vi "ELVIS III v1.0 Build MUX Configuration AO.vi"(11 "AO Channels List":T4) -> (3 "Channel Reservation Info":T1)   [LabVIEW 2021]
uses:
  <vilib>/myRIO/Common/Instrument Driver Framework/myRIO v1.0/AO/typedefs/AO Channels List.ctl
  <vilib>/myRIO/Common/Instrument Driver Framework/myRIO v1.0/AO/typedefs/AO Channels Enum.ctl
  <vilib>/myRIO/Common/Instrument Driver Framework/ELVIS III v1.0/Resource Manager/typedefs/ELVIS III v1.0 Channel Reservation List.ctl
  <vilib>/myRIO/Common/Instrument Driver Framework/ELVIS III v1.0/Resource Manager/typedefs/ELVIS III v1.0 Channel Reservation Info.ctl
  <vilib>/myRIO/Common/Instrument Driver Framework/ELVIS III v1.0/Resource Manager/typedefs/ELVIS III v1.0 Connector List.ctl
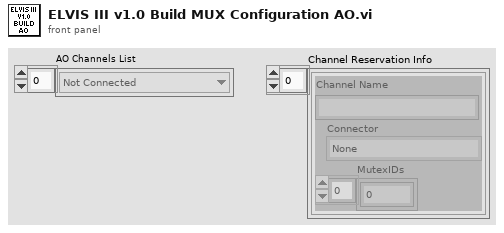
[diagram p1: front panel]
types:
  T1 = typedef "ELVIS III v1.0 Channel Reservation List.ctl" = T2[]
  T2 = typedef "ELVIS III v1.0 Channel Reservation Info.ctl" = cluster{"Channel Name":string, "Connector":T3, "MutexIDs":u32[]}
  T3 = typedef "ELVIS III v1.0 Connector List.ctl" = enum32{"None", "ConnectorA", "ConnectorB"}
  T4 = typedef "AO Channels List.ctl" = T5[]
  T5 = typedef "AO Channels Enum.ctl" = enum16{"Not Connected", "AudioOut/Left", "AudioOut/Right", "C/AO0", "C/AO1", "A/AO0", "A/AO1", "B/AO0", "B/AO1"}
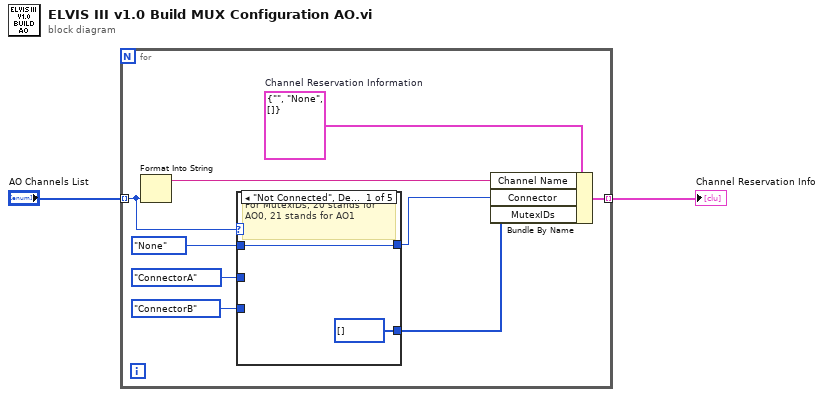
[diagram p0: block diagram]
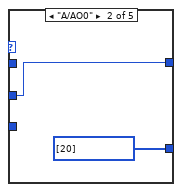
[diagram p2: hidden frame]
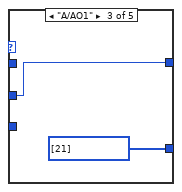
[diagram p3: hidden frame]
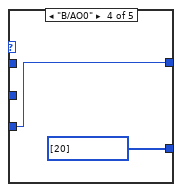
[diagram p4: hidden frame]
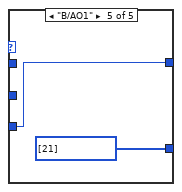
[diagram p5: hidden frame]
diagram:
  n1 = for {
    tunnel: "AO Channels List" -> [w8] mode=indexing
    tunnel: [w9] -> w1 mode=indexing
    w11 = T2 {"Channel Name"="", "Connector"=enum."None", "MutexIDs"=[]}  # Channel Reservation Information
    n2 = Format Into String(w8) -> (resulting string=w10:string)  [unwired: 3 in, 1 out]
    n3 = case shown="\"Not Connected\", Default" w8 {
      tunnel: [i32[] [] i32[] [20] i32[] [21] i32[] [20] i32[] [21]] -> w7
      tunnel: ELVIS_III_v1.0_Connector_List."None" ("Connector") -> [w12 _ _ _ _]
      tunnel: [w12 w14 w16 w19 w21] -> w5
      tunnel: ELVIS_III_v1.0_Connector_List."ConnectorA" ("Connector") -> [_ w14 w16 _ _]
      tunnel: ELVIS_III_v1.0_Connector_List."ConnectorB" ("Connector") -> [_ _ _ w19 w21]
      frame "Not Connected", Default {
        # "For MutexIDs, 20 stands for AO0, 21 stands for AO1"
      }
      frame "A/AO0" {
      }
      frame "A/AO1" {
      }
      frame "B/AO0" {
      }
      frame "B/AO1" {
      }
    }
    n4 = Bundle By Name(cluster=w11, "Channel Name"=w10, "Connector"=w5, "MutexIDs"=w7) -> (w9:T2)
  }
  "Channel Reservation Info" <- w1
